vi "NML Bus Scan Keithley 182.vi"(3 "error out":errorcluster, 4 "String Read In":string, 5 "dup VISA session":refnum<visa-resource-name>) -> (0 "error IO":errorcluster, 1 "String Read Out":string, 2 "VISA Resource Name":refnum<visa-resource-name>)   [LabVIEW 2019]
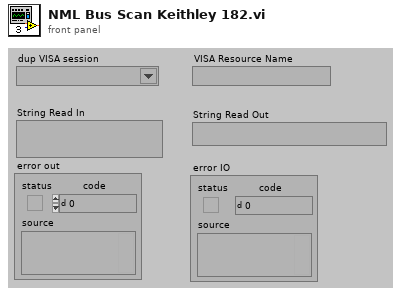
[diagram p1: front panel]
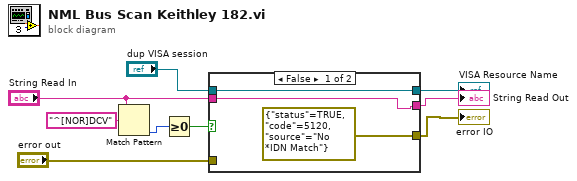
[diagram p0: block diagram]
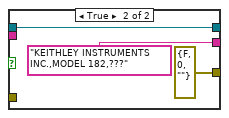
[diagram p2: hidden frame]
diagram:
  n1 = Match Pattern(string="String Read In", regular expression="^[NOR]DCV") -> (offset past match=w1:i32)  [unwired: 1 in, 3 out]
  n2 = Greater Or Equal To 0?(x=w1) -> (x >= 0?=w4:bool)
  n3 = case shown="False" w4 {
    tunnel: [errorcluster {"status"=TRUE, "code"=5120, "source"="No *IDN Match"} ("error out") errorcluster {"status"=FALSE, "code"=0, "source"=""} ("error IO")] -> w9
    tunnel: [w12 "KEITHLEY INSTRUMENTS INC.,MODEL 182,???"] -> w8
    tunnel: [w11 w13] -> w7
    tunnel: "dup VISA session" -> [w11 w13]
    tunnel: "String Read In" -> [w12 _]
    tunnel: "error out" -> [_ _]
    frame False {
    }
    frame True {
    }
  }
  "error IO" <- w9
  "String Read Out" <- w8
  "VISA Resource Name" <- w7
